vi "ACQ Read.vi"(8 "error in (no error)":errorcluster, 11 "Conection Data":T2={"VISA resource name"="COM4"}) -> (0 "error out":errorcluster, 2 "ACQ Data":T1, 3 "Conection Data Out":T2={"VISA resource name"="COM4"})   [LabVIEW 2014, in "SJ-210 Lib.lvlib"]
doc: "Inicia una vez que el VI de status termina de ejecutarse y comienza a consultar los datos que se encuentran en el buffer de la uart. Si la adquisición trae algún error este VI no ejecuta la lectura."
uses:
  SJ-210 Lib.lvlib
  Typedef/Connection Data.ctl
  Typedef/ACQ Data.ctl
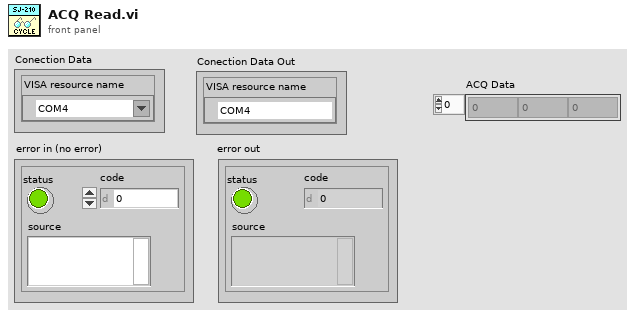
[diagram p1: front panel]
types:
  T1 = typedef "SJ-210 Lib.lvlib/ACQ Data.ctl" = sgl[]
  T2 = typedef "SJ-210 Lib.lvlib/Connection Data.ctl" = cluster{"VISA resource name":refnum<visa-resource-name>}
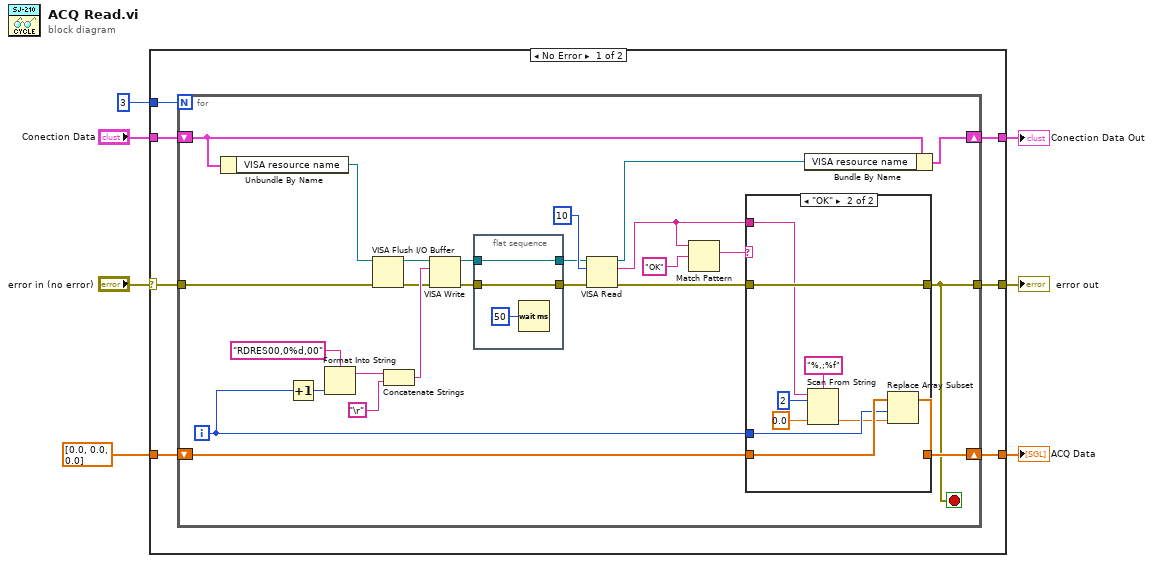
[diagram p0: block diagram]
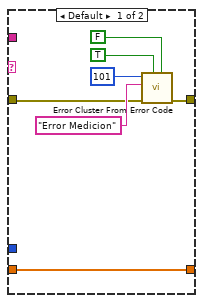
[diagram p2: hidden frame]
diagram:
  n1 = case shown="No Error" "error in (no error)" {
    selector: "error in (no error)" -> [w8 w61]
    tunnel: [w14 w60] -> w7
    tunnel: "Conection Data" -> [w13 w60]
    tunnel: [w12 w61] -> w1
    tunnel: 3 -> [w11 _]
    tunnel: T1 [0.0, 0.0, 0.0] ("ACQ Data") -> [w10 w59]
    tunnel: [w9 w59] -> w3
    frame No Error {
      n2 = for {
        N: w11 -> [_]
        shift-right: [w39] -> w14
        shift-left: w13 -> [w38]
        shift-right: [w27] -> w9
        shift-left: w10 -> [w26]
        tunnel: [w19] -> w12
        tunnel: w8 -> [w24]
        i -> [w25]
        stop <- w19 stop-if-true
        n3 = Unbundle By Name(w38) -> ("VISA resource name"=w29:refnum<visa-resource-name>)
        n4 = Increment(x=w25) -> (x+1=w34:i32)
        n5 = Format Into String(format string="RDRES00,0%d,00", w34) -> (resulting string=w32:string)  [unwired: 2 in, 1 out]
        n6 = VISA Flush I/O Buffer(VISA resource name=w29, error in (no error)=w24) -> (VISA resource name out=w28:refnum<visa-resource-name>, error out=w30:errorcluster)  [unwired: 1 in]
        n7 = Concatenate Strings(w32, "\r") -> (w33:string)
        n8 = VISA Write(VISA resource name=w28, write buffer=w33, error in (no error)=w30) -> (VISA resource name out=w17:refnum<visa-resource-name>, error out=w16:errorcluster)  [unwired: 1 out]
        n9 = flat-sequence {
          tunnel: [w41] -> w18
          tunnel: w17 -> [w41]
          tunnel: w16 -> [w40]
          tunnel: [w40] -> w15
          frame #0 {
            n10 = Wait (ms)(milliseconds to wait=u32 50) -> ()  [unwired: 1 out]
          }
        }
        n11 = VISA Read(VISA resource name=w18, byte count=u32 10, error in (no error)=w15) -> (VISA resource name out=w37:refnum<visa-resource-name>, read buffer=w20:string, error out=w23:errorcluster)  [unwired: 1 out]
        n12 = Match Pattern(string=w20, regular expression="OK") -> (match substring=w21:string)  [unwired: 1 in, 3 out]
        n13 = case shown="\"OK\"" w21 {
          tunnel: [w43 w58] -> w27
          tunnel: w26 -> [w43 w57]
          tunnel: w25 -> [_ w56]
          tunnel: w23 -> [w44 w51]
          tunnel: [w45 w51] -> w19
          tunnel: w20 -> [_ w50]
          frame Default {
            n14 = call <vilib>:"Error Cluster From Error Code.vi"("is warning? (False)"=FALSE, "show call chain? (False)"=TRUE, "error in (no error)"=w44, "error message (\"\")"="Error Medicion" ("error message (\"\")"), "error code (0)"=101) -> ("error out"=w45:errorcluster)  [unwired: 4 in]
          }
          frame "OK" {
            n15 = Scan From String(format string="%,;%f", input string=w50, initial scan location=u32 2, default 1=sgl 0.0 ("default value 1")) -> (output 1=w54:sgl)  [unwired: 1 in, 3 out]
            n16 = Replace Array Subset(array=w57, new element=w54, index=w56) -> (w58:T1)
          }
        }
        n17 = Bundle By Name(cluster=w38, "VISA resource name"=w37) -> (w39:T2)
      }
    }
    frame Error {
    }
  }
  "error out" <- w1
  "Conection Data Out" <- w7
  "ACQ Data" <- w3
